vi "Map.vi"(8 "滑动杆":dbl(slide)=3.0 min=3.0 max=18.0 step=1.0 scale=3.0..18.0, 10 "纬度":string, 11 "经度":string) -> (2 "连接的字符串":string)   [LabVIEW 2018]
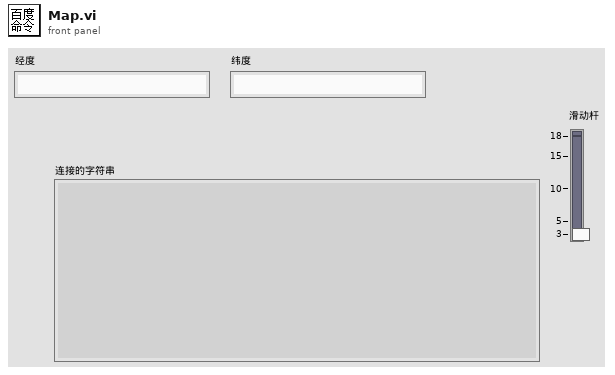
[diagram p1: front panel]
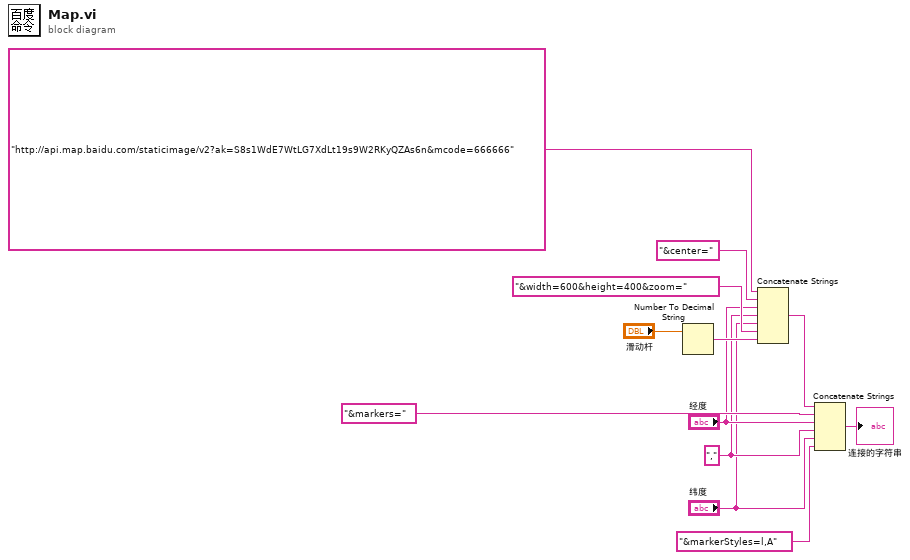
[diagram p0: block diagram]
diagram:
  w5 = ","
  n1 = Number To Decimal String(number="滑动杆") -> (decimal integer string=w8:string)  [unwired: 1 in]
  n2 = Concatenate Strings("http://api.map.baidu.com/staticimage/v2?ak=S8s1WdE7WtLG7XdLt19s9W2RKyQZAs6n&mcode=666666", "&center=" ("字符串"), "经度", w5, "纬度", "&width=600&height=400&zoom=" ("字符串"), w8) -> (w2:string)
  n3 = Concatenate Strings(w2, "&markers=", "经度", w5, "纬度", "&markerStyles=l,A" ("字符串")) -> (→"连接的字符串":string)
